vi "Get Current Step Duration.vi"(8 "error in (no error)":errorcluster, 11 "Output Sequencer in":refnum<class "Output Sequencer.lvclass">) -> (0 "error out":errorcluster, 2 "Duration":dbl, 3 "Output Sequencer out":refnum<class "Output Sequencer.lvclass">)   [LabVIEW 2020, in "Output Sequencer.lvlib" / "Output Sequencer.lvclass"]
uses:
  Output Sequencer.lvclass
  Output Sequencer.lvclass/Output Sequencer.ctl
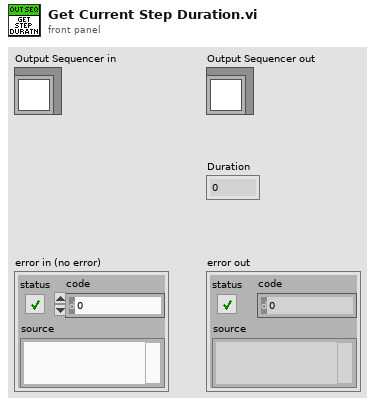
[diagram p1: front panel]
types:
  T1 = typedef "Output Sequencer.lvlib/Output Sequencer.lvclass/Compiled Step.ctl" = cluster{"Precondition":T2, "Duration":dbl, "Mode":string, "Delay Between Values":dbl, "Analog Values":T2[], "Digital Values":T2[], "Postcondition":T2, "On True":string, "On False":string}
  T2 = typedef "Output Sequencer.lvlib/Output Sequencer.lvclass/Expression Data.ctl" = cluster{"Empty?":bool, "Expression":refnum<class "mupExpr.lvclass">, "Variable Names":string[]}
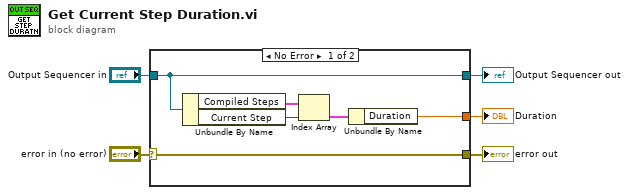
[diagram p0: block diagram]
diagram:
  n1 = case shown="No Error" "error in (no error)" {
    selector: "error in (no error)" -> [w7 w12]
    tunnel: [w11 _] -> w5
    tunnel: "Output Sequencer in" -> [w6 w13]
    tunnel: [w7 w12] -> w2
    tunnel: [w6 w13] -> w1
    frame No Error {
      n2 = Unbundle By Name(w6) -> ("Compiled Steps"=w10:T1[], "Current Step"=w9:i32)
      n3 = Index Array(array=w10, index=w9) -> (element=w8:T1)
      n4 = Unbundle By Name(w8) -> ("Duration"=w11:dbl)
    }
    frame Error {
    }
  }
  "Duration" <- w5
  "error out" <- w2
  "Output Sequencer out" <- w1
